vi "ADC488_Manual_tl.vi"(8 "Clear device prior to command String":bool, 9 "Timeout in msec":i32=1000, 10 "Serial Poll Byte":u8=32, 11 "GPIB Address":T1=8, 12 "Command String":string="u0", 13 "Byte Count Requested":i32=100, 15 "error in (no error)":errorcluster) -> (0 "Status String":string, 1 "Response String":string, 2 "bytes recd.":i32, 4 "error out":errorcluster, 6 "serial poll byte":i16)   [LabVIEW 2010]
uses:
  ADC_GPIB_address.ctl
panel:
  out "readings collected":dbl format="%.2f"
  out "Poll array":bool[](array[boolean])
  # "TRIGGERED"
  # "TRIG ORUN"
  # "BUFF ORUN"
  # "ERROR"
  # "WAITING TRIG"
  # "READY"
  # "SRQ"
  # "COMPLETE"
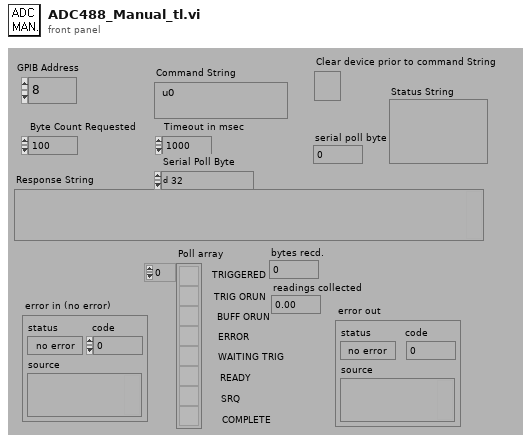
[diagram p1: front panel]
types:
  T1 = typedef "ADC_GPIB_address.ctl" = u8
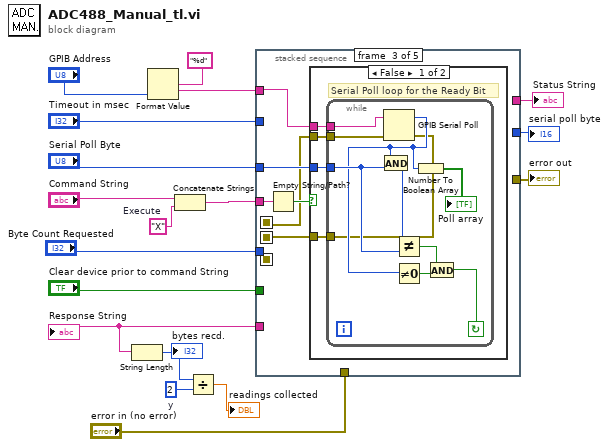
[diagram p0: block diagram]
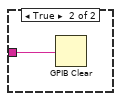
[diagram p3: hidden frame]
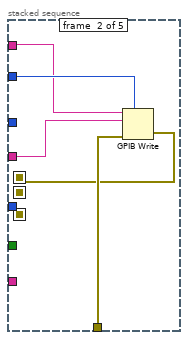
[diagram p4: hidden frame]
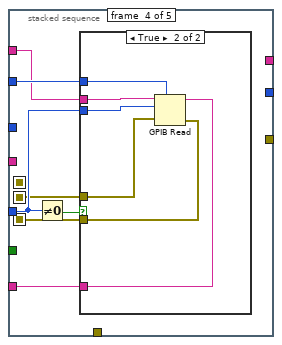
[diagram p6: hidden frame]
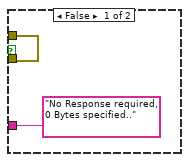
[diagram p7: hidden frame]
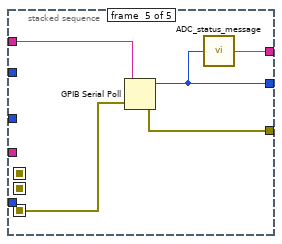
[diagram p8: hidden frame]
diagram:
  w5 = "X"  # Execute
  w8 = 2  # y
  n1 = Format Value(format string="%d", value (0)="GPIB Address") -> (output string=w11:string)  [unwired: 1 out]
  n2 = Concatenate Strings("Command String", w5) -> (w6:string)
  n3 = stacked-sequence {
    seq-local: [_ w22 _ _ _] -> [_ _ w28 _ _]
    seq-local: [_ _ w27 _ _] -> [_ _ _ w49 _]
    seq-local: [_ _ _ w48 _] -> [_ _ _ _ w63]
    tunnel: "Clear device prior to command String" -> [w20 _ _ _ _]
    tunnel: "Timeout in msec" -> [_ w26 _ w52 _]
    tunnel: w6 -> [_ w24 w32 _ _]
    tunnel: "Serial Poll Byte" -> [_ _ w30 _ _]
    tunnel: "Byte Count Requested" -> [_ _ _ w53 _]
    tunnel: [_ _ _ w51 _] -> w10
    tunnel: w11 -> [w19 w25 w29 w50 w67]
    tunnel: [_ _ _ _ w65] -> w4
    tunnel: [_ _ _ _ w66] -> w3
    tunnel: "error in (no error)" -> [_ w23 _ _ _]
    tunnel: [_ _ _ _ w64] -> w1
    frame #0 {
      n4 = case shown="False" w20 {
        tunnel: w19 -> [_ w21]
        frame False {
        }
        frame True {
          n5 = GPIB Clear(3:w21) -> ()  [unwired: 1 in, 2 out]
        }
      }
    }
    frame #1 {
      n6 = GPIB Write(0:w25, 1:w24, 3:w23, 4:w26) -> (6:w22:errorcluster)  [unwired: 2 out]
    }
    frame #2 {
      n7 = Empty String/Path?(string/path=w32) -> (empty?=w31:bool)
      n8 = case shown="False" w31 {
        tunnel: w30 -> [w36 _]
        tunnel: w29 -> [w35 _]
        tunnel: w28 -> [w34 w47]
        tunnel: [w33 w47] -> w27
        frame False {
          # "Serial Poll loop for the Ready Bit"
          n9 = while {
            tunnel: [w37] -> w33
            tunnel: w34 -> [w38]
            tunnel: w35 -> [w43]
            tunnel: w36 -> [w45]
            stop <- w41 continue-if-true
            n10 = GPIB Serial Poll(0:w43, 1:w38) -> (2:w40:i16, 4:w37:errorcluster)  [unwired: 1 out]
            n11 = And(x=w40, y=w45) -> (x .and. y?=w46:i16)
            n12 = Not Equal?(x=w46, y=w45) -> (x != y?=w44:bool)
            n13 = Not Equal To 0?(x=w40) -> (x != 0?=w39:bool)
            n14 = Number To Boolean Array(number=w40) -> (Boolean array=→"Poll array":bool[])
            n15 = And(x=w44, y=w39) -> (x .and. y?=w41:bool)
          }
        }
        frame True {
        }
      }
    }
    frame #3 {
      n16 = Not Equal To 0?(x=w53) -> (x != 0?=w54:bool)
      n17 = case shown="True" w54 {
        tunnel: w53 -> [_ w62]
        tunnel: w52 -> [_ w61]
        tunnel: ["No Response required, 0 Bytes specified.." w60] -> w51
        tunnel: w50 -> [_ w59]
        tunnel: w49 -> [w55 w58]
        tunnel: [w55 w57] -> w48
        frame False {
        }
        frame True {
          n18 = GPIB Read(0:w59, 1:w62, 3:w58, 4:w61) -> (5:w60:string, 7:w57:errorcluster)  [unwired: 2 out]
        }
      }
    }
    frame #4 {
      n19 = GPIB Serial Poll(0:w67, 1:w63) -> (2:w65:i16, 4:w66:errorcluster)  [unwired: 1 out]
      n20 = call "ADC_status_message.vi"("serial poll byte"=w65) -> ("Status String"=w64:string)
    }
  }
  "Response String" <- w10
  "error out" <- w3
  "serial poll byte" <- w4
  "Status String" <- w1
  n21 = String Length(string=w10) -> (length=w9:i32)
  "bytes recd." <- w9
  n22 = Divide(x=w9, y=w8) -> (x/y=→"readings collected":dbl)
